vi "StringEdit.vi"() -> ()   [LabVIEW 2020]
panel:
  out "匹配字符： 1":string
  out "匹配字符后部分：cbar":string
  out "匹配字符前部分： rtS":string
  out "Result2":string
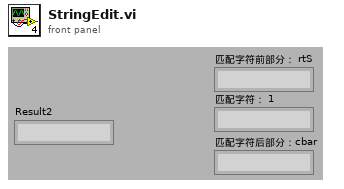
[diagram p1: front panel]
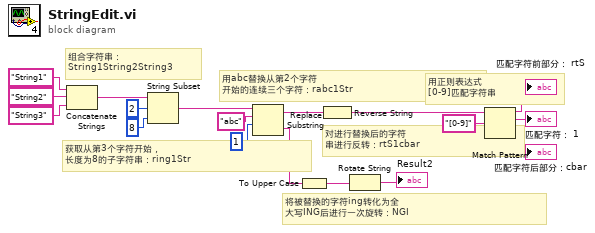
[diagram p0: block diagram]
diagram:
  # "用正则表达式\n[0-9]匹配字符串"
  # "对进行替换后的字符\n串进行反转：rtS1cbar"
  # "将被替换的字符ing转化为全\n大写ING后进行一次旋转：NGI"
  # "用abc替换从第2个字符\n开始的连续三个字符：rabc1Str"
  # "获取从第3个字符开始，\n长度为8的子字符串：ring1Str"
  # "组合字符串：\nString1String2String3"
  n1 = Concatenate Strings("String1" ("string"), "String2" ("string"), "String3" ("string")) -> (w15:string)
  n2 = String Subset(string=w15, offset (0)=2, length (rest)=8 ("length (rest)")) -> (substring=w12:string)
  n3 = Replace Substring(3:1 ("offset (0)"), 4:"abc" ("substring (\"\")"), 5:w12) -> (0:w9:string, 1:w7:string)  [unwired: 1 out]
  n4 = To Upper Case(1:w9) -> (0:w8:string)
  n5 = Reverse String(1:w7) -> (0:w5:string)
  n6 = Rotate String(1:w8) -> (0:→"Result2":string)
  n7 = Match Pattern(string=w5, regular expression="[0-9]") -> (before substring=→"匹配字符前部分： rtS":string, match substring=→"匹配字符： 1":string, after substring=→"匹配字符后部分：cbar":string)  [unwired: 2 out]
